vi "PulseWidth_setup.vi"(1 "Signal-high duration":u32=20, 2 "Signal-high lead-up":u32=10) -> (0 "Error output":T1)   [LabVIEW 2010]
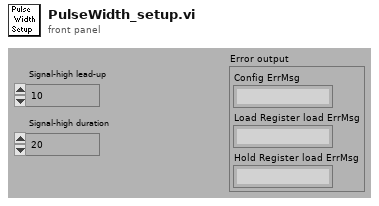
[diagram p1: front panel]
types:
  T1 = cluster{"Config ErrMsg":string, "Load Register load ErrMsg":string, "Hold Register load ErrMsg":string}
  T2 = cluster{"ErrMsg":string, "ErrMsg":string, "ErrMsg":string}
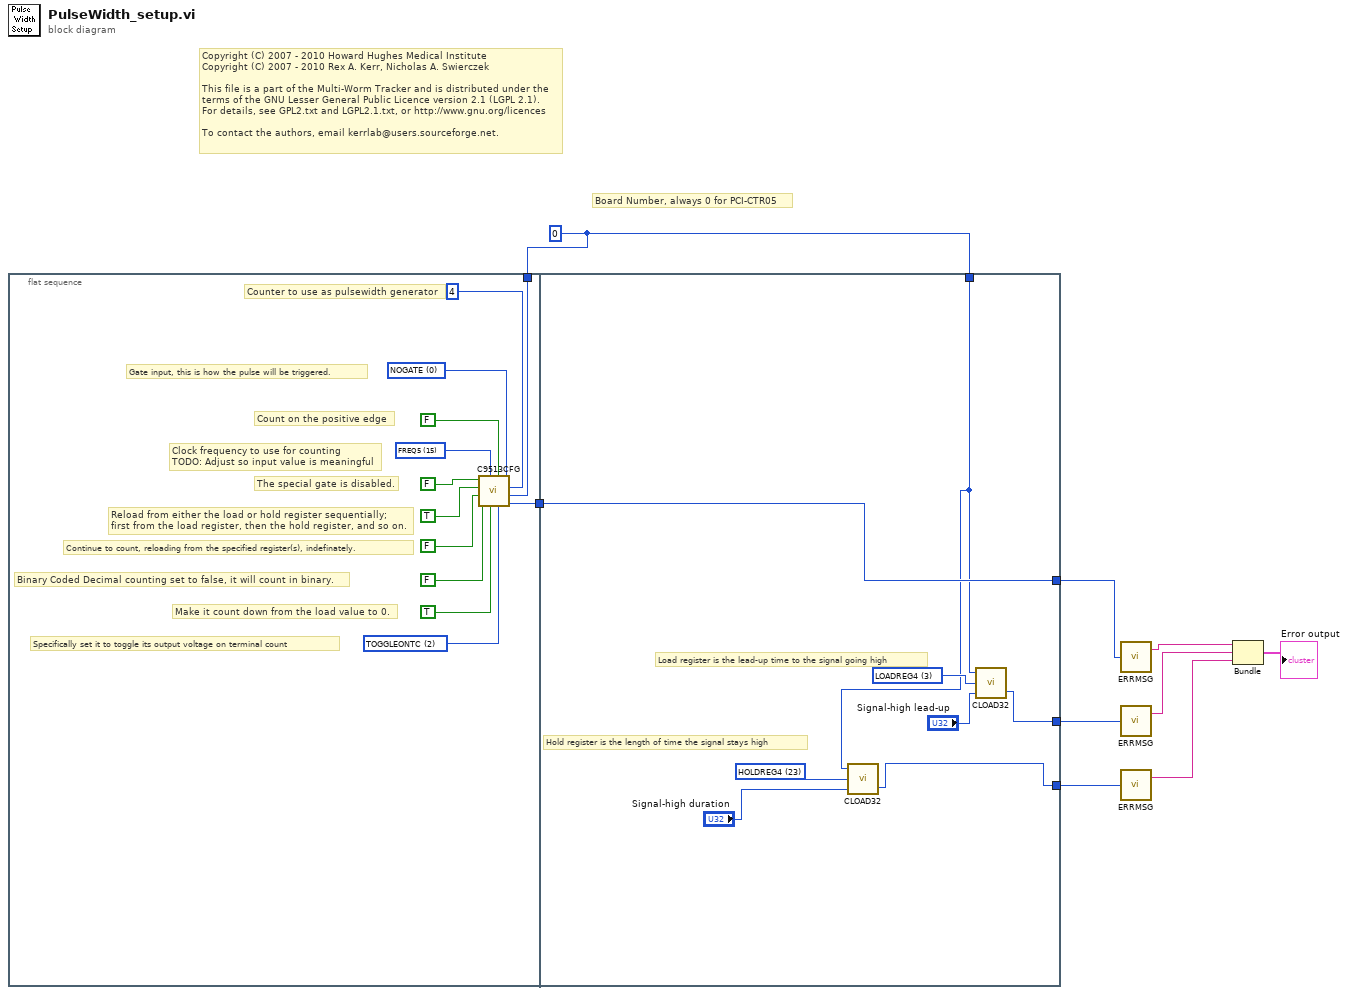
[diagram p0: block diagram]
diagram:
  w1 = u32 0 ("BoardNum (0)")
  # "Copyright (C) 2007 - 2010 Howard Hughes Medical Institute\nCopyright (C) 2007 - 2010 Rex A. Kerr, Nicholas A. Swierczek\n \nThis file is a part of the Multi-Worm Tracker and is distributed under the\nterms of the GNU Lesser General Public Licence version 2.1 (LGPL 2.1).\nFor details, see GPL2.txt and LGPL2.1.txt, or http://www.gnu.org/licences\n \nTo contact the authors, email kerrlab@users.sourceforge.net."
  # "Board Number, always 0 for PCI-CTR05"
  n1 = flat-sequence {
    tunnel: [w11] -> w2
    tunnel: w1 -> [w10]
    tunnel: [w25] -> w5
    tunnel: [w24] -> w4
    tunnel: [w23] -> w3
    tunnel: w2 -> [w23]
    tunnel: w1 -> [w22]
    frame #0 {
      w12 = u32 2 items=["ALWAYSLOW", "HIGHPULSEONTC", "TOGGLEONTC", "DISCONNECTED", "LOWPULSEONTC"] ("OutputControl (LOW)")
      w18 = u32 15 items=["TCPREVCTR", "CTRINPUT1", "CTRINPUT2", "CTRINPUT3", "CTRINPUT4", "CTRINPUT5", "GATE1", "GATE2", "GATE3", "GATE4", "GATE5", "FREQ1", "FREQ2", "FREQ3", "FREQ4", "FREQ5", "CTRINPUT6", "CTRINPUT7", "CTRINPUT8", "CTRINPUT9", "CTRINPUT10", "GATE6", "GATE7", "GATE8", "GATE9", "GATE10", "FREQ6", "FREQ7", "FREQ8", "FREQ9", "FREQ10", "CTRINPUT11", "CTRINPUT12", "CTRINPUT13", "CTRINPUT14", "CTRINPUT15", "GATE11", "GATE12", "GATE13", "GATE14", "GATE15", "FREQ11", "FREQ12", "FREQ13", "FREQ14", "FREQ15", "CTRINPUT16", "CTRINPUT17", "CTRINPUT18", "CTRINPUT19", "CTRINPUT20", "GATE16", "GATE17", "GATE18", "GATE19", "GATE20", "FREQ16", "FREQ17", "FREQ18", "FREQ19", "FREQ20"] ("CountSource")
      w20 = u32 0 items=["NOGATE", "AHLTCPREVCTR", "AHLNEXTGATE", "AHLPREVGATE", "AHLGATE", "ALLGATE", "AHEGATE", "ALEGATE"] ("GateControl")
      # "Continue to count, reloading from the specified register(s), indefinately."
      # "Specifically set it to toggle its output voltage on terminal count"
      # "Make it count down from the load value to 0."
      # "Binary Coded Decimal counting set to false, it will count in binary."
      # "Reload from either the load or hold register sequentially;\nfirst from the load register, then the hold register, and so on."
      # "The special gate is disabled."
      # "Clock frequency to use for counting\nTODO: Adjust so input value is meaningful"
      # "Count on the positive edge"
      # "Gate input, this is how the pulse will be triggered."
      # "Counter to use as pulsewidth generator"
      n2 = call <menus>:"C9513CFG.VI"("BCDMode (DISABLED)"=FALSE, "CountDirection (UP)"=TRUE, "OutputControl (LOW)"=w12, "Recycle (ONETIME)"=FALSE, "BoardNum (0)"=w10, "Reload (LOADREG)"=TRUE, "CounterNum (1)"=u32 4 ("CounterNum"), "SpecialGate (DISABLED)"=FALSE, "CountSource"=w18, "CountEdge(POSITIVE)"=FALSE, "GateControl"=w20) -> ("ErrCode"=w11:i32)
    }
    frame #1 {
      w28 = u32 3 items=["LOADREG1", "LOADREG2", "LOADREG3", "LOADREG4", "LOADREG5", "LOADREG6", "LOADREG7", "LOADREG8", "LOADREG9", "LOADREG10", "LOADREG11", "LOADREG12", "LOADREG13", "LOADREG14", "LOADREG15", "LOADREG16", "LOADREG17", "LOADREG18", "LOADREG19", "LOADREG20", "HOLDREG1", "HOLDREG2", "HOLDREG3", "HOLDREG4", "HOLDREG5", "HOLDREG6", "HOLDREG7", "HOLDREG8", "HOLDREG9", "HOLDREG10", "HOLDREG11", "HOLDREG12", "HOLDREG13", "HOLDREG14", "HOLDREG15", "HOLDREG16", "HOLDREG17", "HOLDREG18", "HOLDREG19", "HOLDREG20", "ALARM1CHIP1", "ALARM2CHIP1", "ALARM1CHIP2", "ALARM2CHIP2", "ALARM1CHIP3", "ALARM2CHIP3", "ALARM1CHIP4", "ALARM2CHIP4", "COUNT1", "COUNT2", "COUNT3", "COUNT4", "PRESET1", "PRESET2", "PRESET3", "PRESET4", "PRESCALER1", "PRESCALER2", "PRESCALER3", "PRESCALER4"] ("Counter 1 Load RegName")
      w26 = u32 23 items=["LOADREG1", "LOADREG2", "LOADREG3", "LOADREG4", "LOADREG5", "LOADREG6", "LOADREG7", "LOADREG8", "LOADREG9", "LOADREG10", "LOADREG11", "LOADREG12", "LOADREG13", "LOADREG14", "LOADREG15", "LOADREG16", "LOADREG17", "LOADREG18", "LOADREG19", "LOADREG20", "HOLDREG1", "HOLDREG2", "HOLDREG3", "HOLDREG4", "HOLDREG5", "HOLDREG6", "HOLDREG7", "HOLDREG8", "HOLDREG9", "HOLDREG10", "HOLDREG11", "HOLDREG12", "HOLDREG13", "HOLDREG14", "HOLDREG15", "HOLDREG16", "HOLDREG17", "HOLDREG18", "HOLDREG19", "HOLDREG20", "ALARM1CHIP1", "ALARM2CHIP1", "ALARM1CHIP2", "ALARM2CHIP2", "ALARM1CHIP3", "ALARM2CHIP3", "ALARM1CHIP4", "ALARM2CHIP4", "COUNT1", "COUNT2", "COUNT3", "COUNT4", "PRESET1", "PRESET2", "PRESET3", "PRESET4", "PRESCALER1", "PRESCALER2", "PRESCALER3", "PRESCALER4"] ("Counter 1 Hold RegName")
      # "Load register is the lead-up time to the signal going high"
      # "Hold register is the length of time the signal stays high"
      n3 = call <menus>:"CLOAD32.VI"("LoadValue"="Signal-high duration", "RegName"=w26, "BoardNum (0)"=w22) -> ("ErrCode"=w24:i32)  [unwired: 1 out]
      n4 = call <menus>:"CLOAD32.VI"("LoadValue"="Signal-high lead-up", "RegName"=w28, "BoardNum (0)"=w22) -> ("ErrCode"=w25:i32)  [unwired: 1 out]
    }
  }
  n5 = call <menus>:"ERRMSG.VI"("ErrCode"=w3) -> ("ErrMsg"=w9:string)  [unwired: 1 out]
  n6 = call <menus>:"ERRMSG.VI"("ErrCode"=w5) -> ("ErrMsg"=w8:string)  [unwired: 1 out]
  n7 = call <menus>:"ERRMSG.VI"("ErrCode"=w4) -> ("ErrMsg"=w7:string)  [unwired: 1 out]
  n8 = Bundle("ErrMsg"=w9, "ErrMsg"=w8, "ErrMsg"=w7) -> (→"Error output":T2)  [unwired: 1 in]
